vi "Aktualizacja listy z punktami do usunięcia -dane z dwoch kolumn.vi"(7 "1 kolumna":bool=TRUE, 8 "text add 2":i32, 9 "text add 1":i32, 10 "Lista współrzędnych":string[][](array[string]), 11 "Lista z punktami do usunięcia":refnum<vi>) -> ()   [LabVIEW 2015, in "Biblioteka moduł map v3.lvlib" / "Obsługa listy współrzędnych.lvlib"]
doc: "Dodanie do kontrolki enumerate nazw wszystkich punktów znajdujących sie na liście współrzędnych."
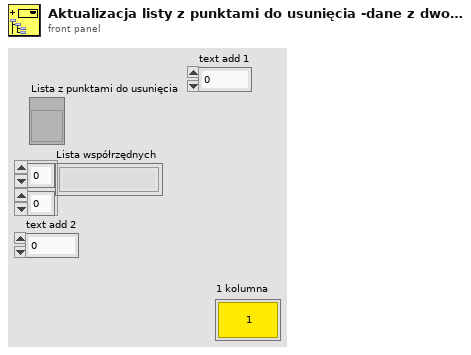
[diagram p1: front panel]
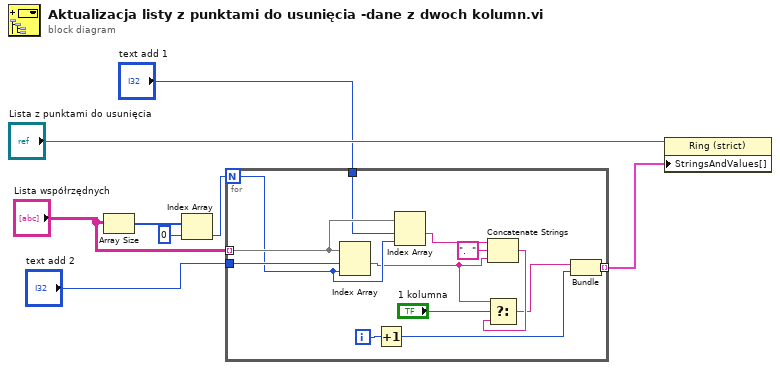
[diagram p0: block diagram]
diagram:
  n1 = Array Size(array="Lista współrzędnych") -> (size(s)=w6:i32[])
  n2 = Index Array(array=w6, index=0) -> (element=w4:i32)
  n3 = for {
    N: w4 -> [w16]
    tunnel: "Lista współrzędnych" -> [w17] mode=indexing
    tunnel: [w21] -> w3 mode=indexing
    tunnel: "text add 2" -> [w18]
    tunnel: "text add 1" -> [w15]
    i -> [w20]
    n4 = Index Array(array=w17, index #1=w18, index #2=w16) -> (element #1=w11:string)  [unwired: 1 out]
    n5 = Increment(x=w20) -> (x+1=w19:i32)
    n6 = Index Array(array=w17, index #1=w15, index #2=w16) -> (element #1=w14:string)  [unwired: 1 out]
    n7 = Concatenate Strings(w14, ".  " ("string"), w11) -> (w10:string)
    n8 = Select(t=w11, s="1 kolumna", f=w10) -> (s? t:f=w9:string)
    n9 = Bundle(w9, w19) -> (w21:cluster{string, i32})  [unwired: 1 in]
  }
  n10 = property class="Ring (strict)"(reference="Lista z punktami do usunięcia", "StringsAndValues[]"=w3) -> ()  [unwired: 1 in, 2 out]
